vi "NicmosWriteFilter.vi"(3 "refnum in":T1, 9 "error in (no error)":errorcluster) -> (0 "refnum out":T1, 6 "error out":errorcluster)   [LabVIEW 2009]
uses:
  <vilib>/Utility/config.llb/Config Data RefNum.ctl
  <vilib>/Utility/config.llb/NI_LVConfig.lvlib
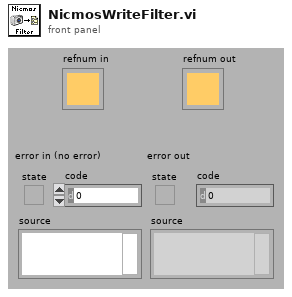
[diagram p1: front panel]
types:
  T1 = typedef "NI_LVConfig.lvlib/Config Data RefNum.ctl" = refnum<k1>
  T2 = typedef "NICMOS.FILTER.ctl" = string
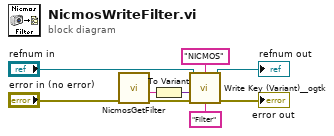
[diagram p0: block diagram]
diagram:
  n1 = call "NicmosGetFilter.vi"("error in (no error)"="error in (no error)") -> ("FILTER out"=w5:T2, "error out"=w6:errorcluster)  [unwired: 7 in]
  n2 = To Variant(anything=w5) -> (Variant=w9:variant)
  n3 = call <userlib>:"Write Key (Variant)__ogtk.vi"("section"="NICMOS", "error in (no error)"=w6, "key-value"=w9, "key (optional)"="Filter", "refnum"="refnum in") -> ("error out"=→"error out":errorcluster, "refnum out"=→"refnum out":T1)  [unwired: 5 in]
